vi "DEMO_04_WAVE_PRO.vi"() -> ()   [LabVIEW 2014]
uses:
  <vilib>/Instr/_visa.llb/VISA Configure Serial Port (Instr).vi
panel:
  in  "开始":bool
  in  "发送数据 3":bool
  in  "发送数据 2":bool
  in  "相位角 3":dbl
  in  "幅值 3":dbl
  in  "偏移 3":dbl
  in  "相位角 2":dbl
  in  "幅值 2":dbl
  in  "偏移 2":dbl
  in  "相位角":dbl
  in  "打开串口":bool
  in  "上位机控制":bool
  in  "停止传送":bool
  in  "开闭环":u16(ring) items=["  开环", "  闭环"]
  in  "幅值":dbl
  in  "频率":dbl
  in  "偏移":dbl
  in  "波形选择":u16(ring) items=["正弦波", "矩形波", "三角波", "锯齿波"]
  in  "发送数据":bool
  in  "波特率":u32(ring)=9600 items=["75"=75, "110"=110, "134"=134, "150"=150, "300"=300, "600"=600, "1200"=1200, "1800"=1800, "2400"=2400, "4800"=4800, "7200"=7200, "9600"=9600, "14400"=14400, "19200"=19200, "28800"=28800, "38400"=38400, "56000"=56000, "57600"=57600, "115200"=115200, "128000"=128000, "230400"=230400]
  in  "奇偶":enum16{"None", "Odd", "Even", "Mark", "Space"}(ring) caption="校验"
  in  "VISA资源名称":refnum<visa-resource-name>="COM1"
  # "发送相位角波形"
  # "下位机开闭环需要统一"
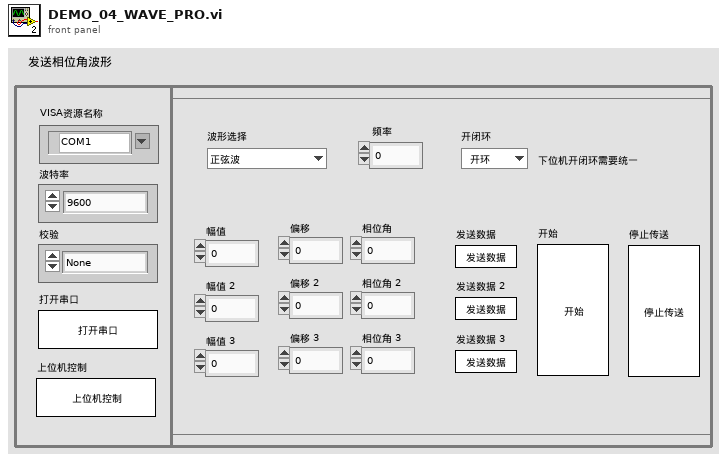
[diagram p1: front panel]
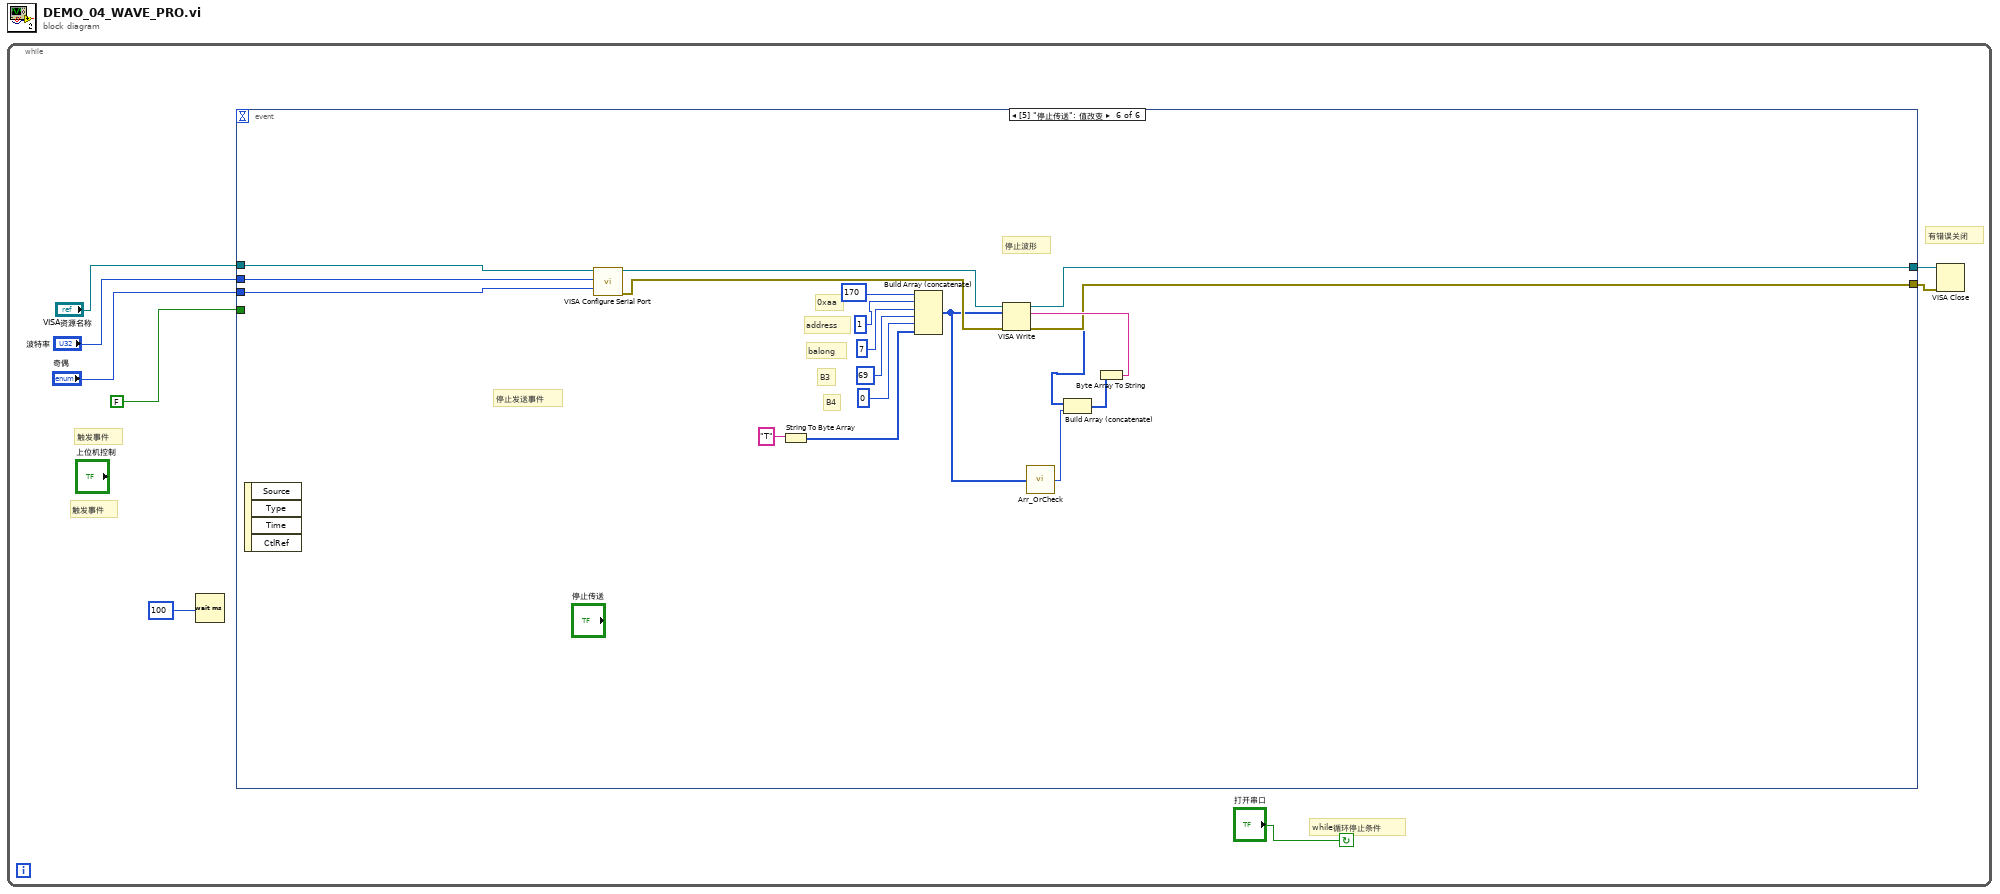
[diagram p0: block diagram]
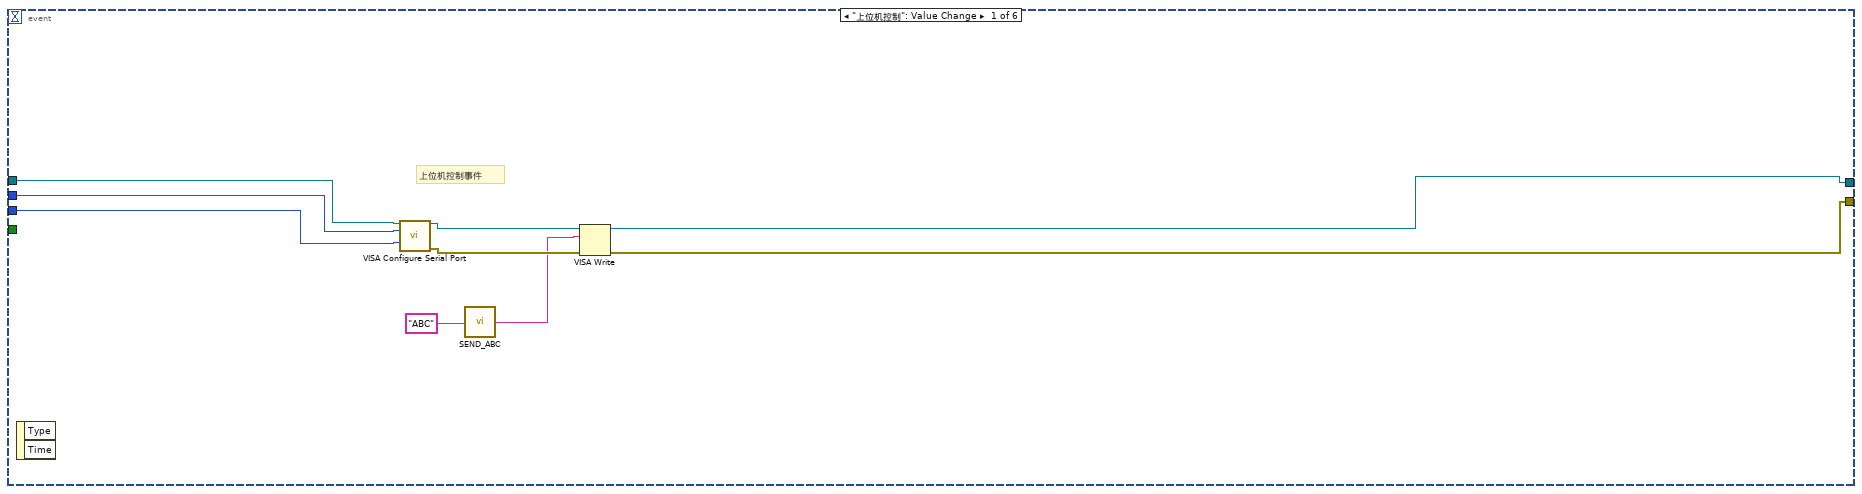
[diagram p2: hidden frame]
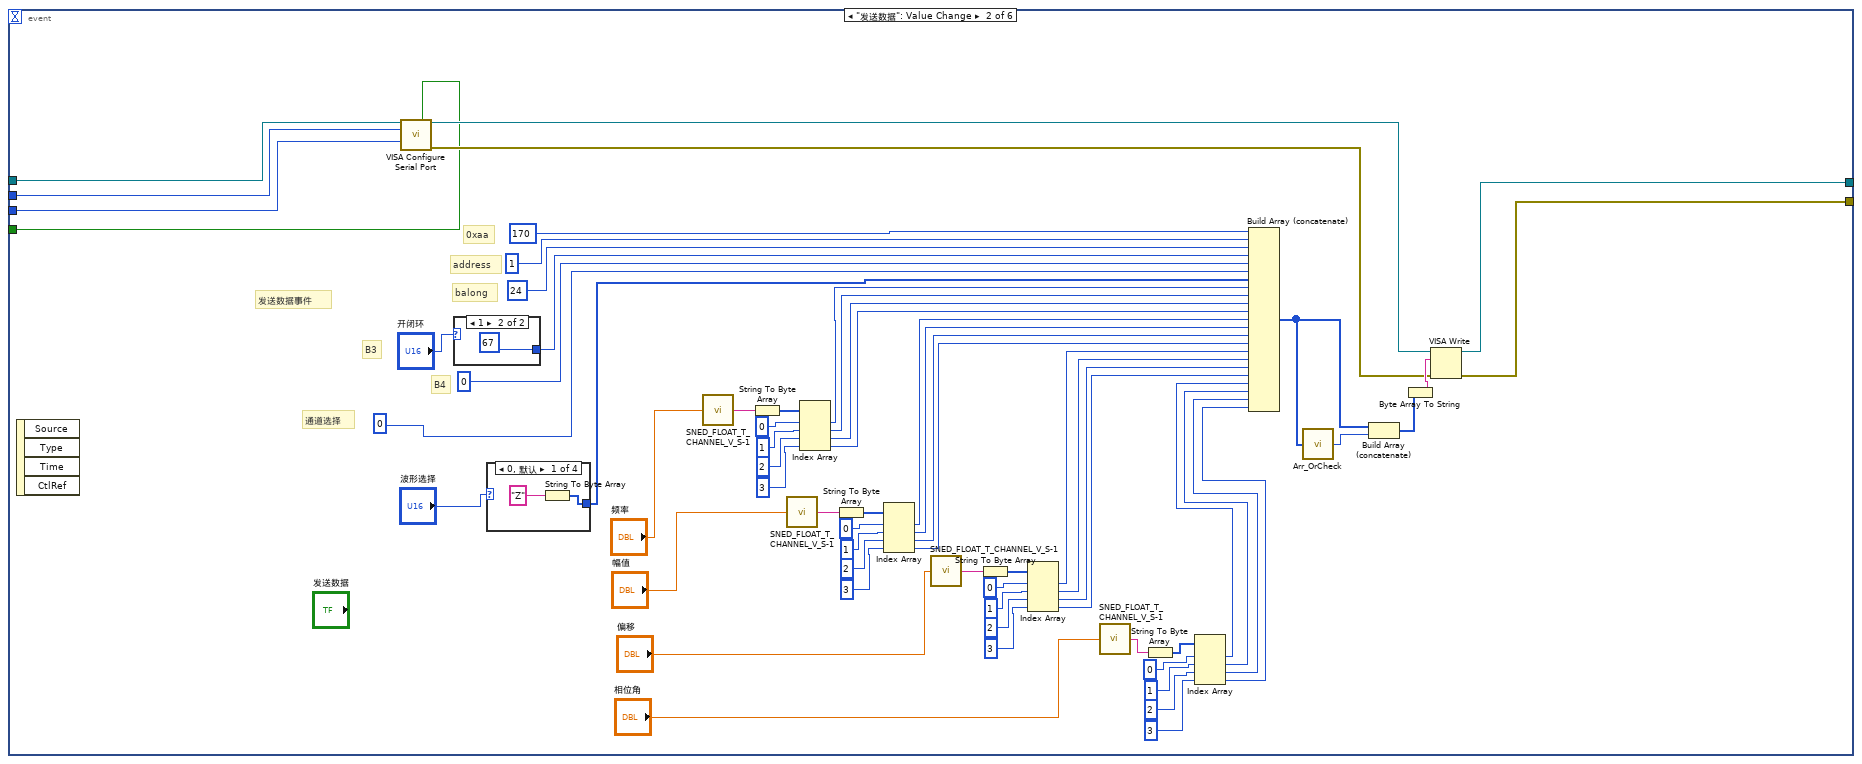
[diagram p3: hidden frame]
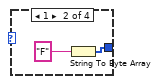
[diagram p4: hidden frame]
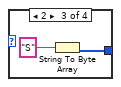
[diagram p5: hidden frame]
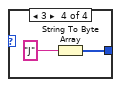
[diagram p6: hidden frame]
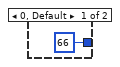
[diagram p7: hidden frame]
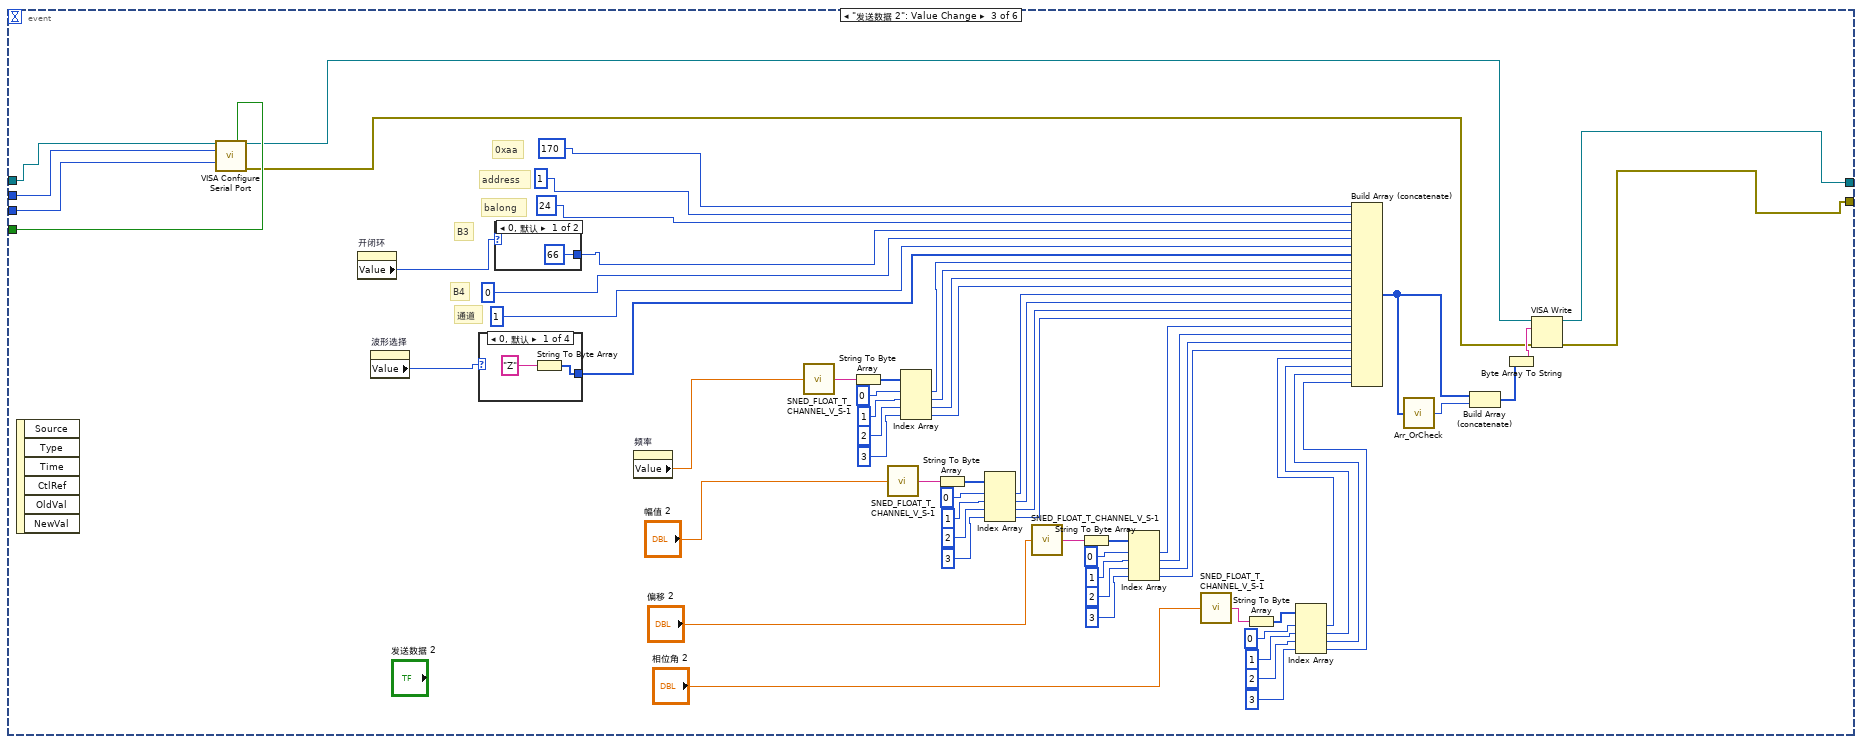
[diagram p8: hidden frame]
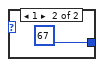
[diagram p9: hidden frame]
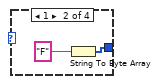
[diagram p10: hidden frame]
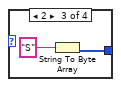
[diagram p11: hidden frame]
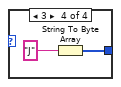
[diagram p12: hidden frame]
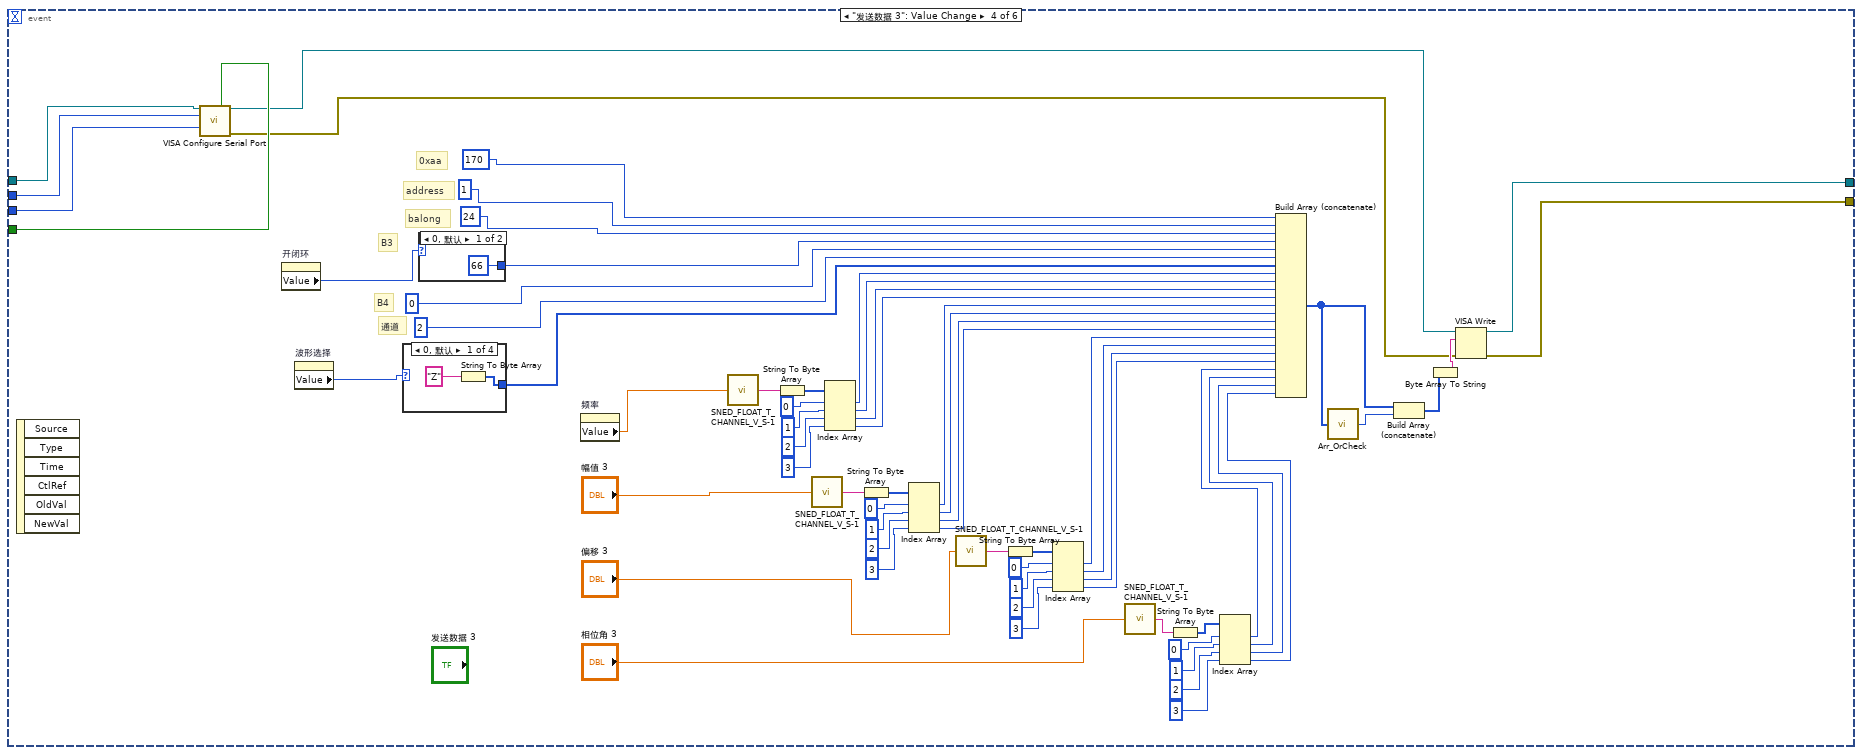
[diagram p13: hidden frame]
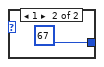
[diagram p14: hidden frame]
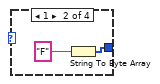
[diagram p15: hidden frame]
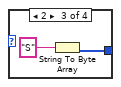
[diagram p16: hidden frame]
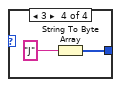
[diagram p17: hidden frame]
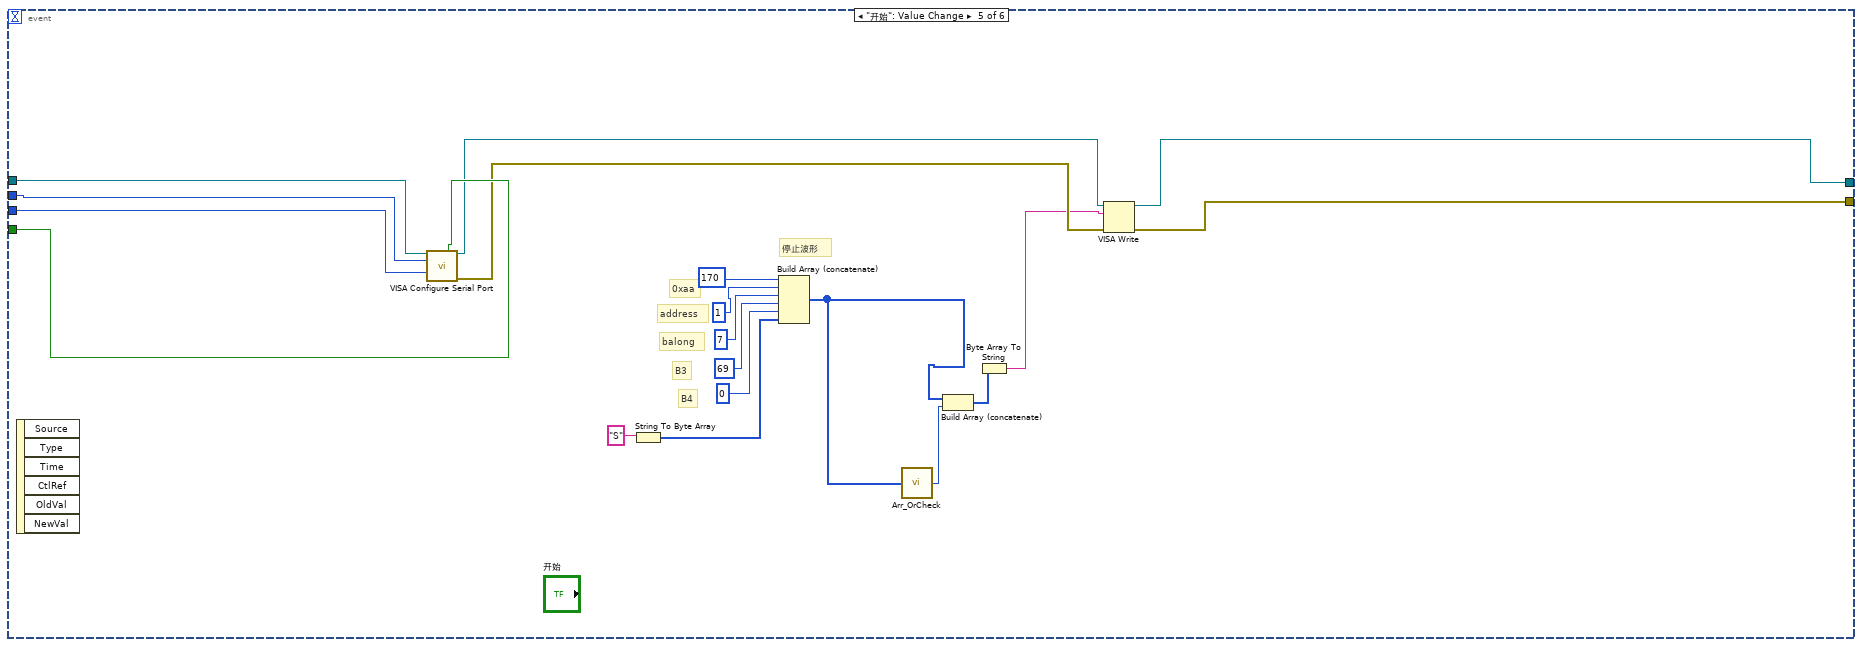
[diagram p18: hidden frame]
diagram:
  n1 = while {
    stop <- "打开串口" continue-if-true
    # "有错误关闭"
    # "while循环停止条件"
    # "触发事件"
    # "触发事件"
    n2 = Wait (ms)(milliseconds to wait=100) -> ()  [unwired: 1 out]
    n3 = event shown="[5] \"停止传送\": 值改变" {
      selector: _ -> [_ _ _ _ _ _]
      dyn-events: _ -> [_ _ _ _ _ _]
      timeout: _ -> [_ _ _ _ _ _]
      tunnel: "VISA资源名称" -> [w17 w35 w101 w177 w252 w279]
      tunnel: "波特率" -> [w16 w34 w100 w176 w251 w278]
      tunnel: "奇偶" -> [w15 w33 w99 w175 w250 w277]
      tunnel: [w10 w21 w94 w170 w245 w266] -> w3
      tunnel: [w9 w20 w95 w171 w244 w265] -> w2
      tunnel: FALSE -> [_ w19 w98 w174 w249 _]
      event "上位机控制": Value Change {
        # "上位机控制事件"
        n4 = event-data() -> ()  [unwired: 1 in, 2 out]
        n5 = call-poly "VISA Configure Serial Port"("VISA resource name"=w17, "baud rate (9600)"=w16, "parity (0:none)"=w15) -> ("VISA resource name out"=w14:refnum<visa-resource-name>, "error out"=w13:errorcluster)  [unwired: 11 in]
        n6 = call "SEND_ABC.vi"("SEND_ARR"="ABC") -> ("SEND_CHR"=w11:string)
        n7 = VISA Write(VISA resource name=w14, write buffer=w11, error in (no error)=w13) -> (VISA resource name out=w10:refnum<visa-resource-name>, error out=w9:errorcluster)  [unwired: 1 out]
      }
      event "发送数据": Value Change {
        # "通道选择"
        # "B4"
        # "B3"
        # "balong"
        # "address"
        # "0xaa"
        # "发送数据事件"
        n8 = event-data() -> ()  [unwired: 1 in, 4 out]
        n9 = call-poly "VISA Configure Serial Port"("VISA resource name"=w35, "Enable Termination\nChar (T)"=w19, "baud rate (9600)"=w34, "parity (0:none)"=w33) -> ("VISA resource name out"=w37:refnum<visa-resource-name>, "error out"=w36:errorcluster)  [unwired: 10 in]
        n10 = case shown="1" "开闭环" {
          tunnel: [66 67] -> w60
          frame 0, Default {
          }
          frame 1 {
          }
        }
        n11 = case shown="0, 默认" "波形选择" {
          tunnel: [w83 w85 w87 w89] -> w58
          frame 0, Default {
            n12 = String To Byte Array(string="Z") -> (unsigned byte array=w83:u8[])
          }
          frame 1 {
            n13 = String To Byte Array(string="F") -> (unsigned byte array=w85:u8[])
          }
          frame 2 {
            n14 = String To Byte Array(string="S") -> (unsigned byte array=w87:u8[])
          }
          frame 3 {
            n15 = String To Byte Array(string="J") -> (unsigned byte array=w89:u8[])
          }
        }
        n16 = call "SNED_FLOAT_T_CHANNEL_V_S-1.vi"("数据"="频率") -> ("字符串"=w81:string)
        n17 = String To Byte Array(string=w81) -> (unsigned byte array=w80:u8[])
        n18 = call "SNED_FLOAT_T_CHANNEL_V_S-1.vi"("数据"="幅值") -> ("字符串"=w75:string)
        n19 = Index Array(array=w80, index #1=0, index #2=1, index #3=2, index #4=3) -> (element #1=w54:u8, element #2=w53:u8, element #3=w52:u8, element #4=w51:u8)
        n20 = String To Byte Array(string=w75) -> (unsigned byte array=w74:u8[])
        n21 = Index Array(array=w74, index #1=0, index #2=1, index #3=2, index #4=3) -> (element #1=w50:u8, element #2=w49:u8, element #3=w48:u8, element #4=w47:u8)
        n22 = call "SNED_FLOAT_T_CHANNEL_V_S-1.vi"("数据"="偏移") -> ("字符串"=w69:string)
        n23 = String To Byte Array(string=w69) -> (unsigned byte array=w68:u8[])
        n24 = Index Array(array=w68, index #1=0, index #2=1, index #3=2, index #4=3) -> (element #1=w46:u8, element #2=w45:u8, element #3=w44:u8, element #4=w43:u8)
        n25 = call "SNED_FLOAT_T_CHANNEL_V_S-1.vi"("数据"="相位角") -> ("字符串"=w31:string)
        n26 = String To Byte Array(string=w31) -> (unsigned byte array=w30:u8[])
        n27 = Index Array(array=w30, index #1=0, index #2=1, index #3=2, index #4=3) -> (element #1=w25:u8, element #2=w24:u8, element #3=w23:u8, element #4=w22:u8)
        n28 = Build Array (concatenate)(170, 1, 24, w60, 0, 0, w58, w54, w53, w52, w51, w50, w49, w48, w47, w46, w45, w44, w43, w25, w24, w23, w22) -> (w42:i32[])
        n29 = call "Arr_OrCheck.vi"("数组"=w42) -> ("抑或的数据值"=w41:u8)
        n30 = Build Array (concatenate)(w42, w41) -> (w40:i32[])
        n31 = Byte Array To String(unsigned byte array=w40) -> (string=w39:string)
        n32 = VISA Write(VISA resource name=w37, write buffer=w39, error in (no error)=w36) -> (VISA resource name out=w21:refnum<visa-resource-name>, error out=w20:errorcluster)  [unwired: 1 out]
      }
      event "发送数据 2": Value Change {
        # "通道"
        # "B4"
        # "B3"
        # "balong"
        # "address"
        # "0xaa"
        n33 = event-data() -> ()  [unwired: 1 in, 6 out]
        n34 = call-poly "VISA Configure Serial Port"("VISA resource name"=w101, "Enable Termination\nChar (T)"=w98, "baud rate (9600)"=w100, "parity (0:none)"=w99) -> ("VISA resource name out"=w97:refnum<visa-resource-name>, "error out"=w96:errorcluster)  [unwired: 10 in]
        n35 = property on="开闭环" class="Ring (严格)"() -> ("Value"=w113:u16)  [unwired: 2 in, 2 out]
        n36 = property on="波形选择" class="Ring (严格)"() -> ("Value"=w112:u16)  [unwired: 2 in, 2 out]
        n37 = case shown="0, 默认" w112 {
          tunnel: [w160 w162 w164 w166] -> w111
          frame 0, Default {
            n38 = String To Byte Array(string="Z") -> (unsigned byte array=w160:u8[])
          }
          frame 1 {
            n39 = String To Byte Array(string="F") -> (unsigned byte array=w162:u8[])
          }
          frame 2 {
            n40 = String To Byte Array(string="S") -> (unsigned byte array=w164:u8[])
          }
          frame 3 {
            n41 = String To Byte Array(string="J") -> (unsigned byte array=w166:u8[])
          }
        }
        n42 = case shown="0, 默认" w113 {
          tunnel: [66 67] -> w108
          frame 0, Default {
          }
          frame 1 {
          }
        }
        n43 = property on="频率" class="DigNum (严格)"() -> ("Value"=w93:dbl)  [unwired: 2 in, 2 out]
        n44 = call "SNED_FLOAT_T_CHANNEL_V_S-1.vi"("数据"=w93) -> ("字符串"=w157:string)
        n45 = String To Byte Array(string=w157) -> (unsigned byte array=w156:u8[])
        n46 = call "SNED_FLOAT_T_CHANNEL_V_S-1.vi"("数据"="幅值 2") -> ("字符串"=w151:string)
        n47 = Index Array(array=w156, index #1=0, index #2=1, index #3=2, index #4=3) -> (element #1=w139:u8, element #2=w138:u8, element #3=w137:u8, element #4=w136:u8)
        n48 = String To Byte Array(string=w151) -> (unsigned byte array=w150:u8[])
        n49 = Index Array(array=w150, index #1=0, index #2=1, index #3=2, index #4=3) -> (element #1=w135:u8, element #2=w134:u8, element #3=w133:u8, element #4=w132:u8)
        n50 = call "SNED_FLOAT_T_CHANNEL_V_S-1.vi"("数据"="偏移 2") -> ("字符串"=w145:string)
        n51 = String To Byte Array(string=w145) -> (unsigned byte array=w144:u8[])
        n52 = Index Array(array=w144, index #1=0, index #2=1, index #3=2, index #4=3) -> (element #1=w131:u8, element #2=w130:u8, element #3=w129:u8, element #4=w128:u8)
        n53 = call "SNED_FLOAT_T_CHANNEL_V_S-1.vi"("数据"="相位角 2") -> ("字符串"=w123:string)
        n54 = String To Byte Array(string=w123) -> (unsigned byte array=w122:u8[])
        n55 = Index Array(array=w122, index #1=0, index #2=1, index #3=2, index #4=3) -> (element #1=w117:u8, element #2=w116:u8, element #3=w115:u8, element #4=w114:u8)
        n56 = Build Array (concatenate)(170, 1, 24, w108, 0, 1, w111, w139, w138, w137, w136, w135, w134, w133, w132, w131, w130, w129, w128, w117, w116, w115, w114) -> (w127:i32[])
        n57 = call "Arr_OrCheck.vi"("数组"=w127) -> ("抑或的数据值"=w126:u8)
        n58 = Build Array (concatenate)(w127, w126) -> (w125:i32[])
        n59 = Byte Array To String(unsigned byte array=w125) -> (string=w124:string)
        n60 = VISA Write(VISA resource name=w97, write buffer=w124, error in (no error)=w96) -> (VISA resource name out=w94:refnum<visa-resource-name>, error out=w95:errorcluster)  [unwired: 1 out]
      }
      event "发送数据 3": Value Change {
        # "通道"
        # "B4"
        # "B3"
        # "balong"
        # "address"
        # "0xaa"
        n61 = event-data() -> ()  [unwired: 1 in, 6 out]
        n62 = call-poly "VISA Configure Serial Port"("VISA resource name"=w177, "Enable Termination\nChar (T)"=w174, "baud rate (9600)"=w176, "parity (0:none)"=w175) -> ("VISA resource name out"=w173:refnum<visa-resource-name>, "error out"=w172:errorcluster)  [unwired: 10 in]
        n63 = property on="开闭环" class="Ring (严格)"() -> ("Value"=w189:u16)  [unwired: 2 in, 2 out]
        n64 = property on="波形选择" class="Ring (严格)"() -> ("Value"=w188:u16)  [unwired: 2 in, 2 out]
        n65 = case shown="0, 默认" w188 {
          tunnel: [w235 w237 w239 w241] -> w187
          frame 0, Default {
            n66 = String To Byte Array(string="Z") -> (unsigned byte array=w235:u8[])
          }
          frame 1 {
            n67 = String To Byte Array(string="F") -> (unsigned byte array=w237:u8[])
          }
          frame 2 {
            n68 = String To Byte Array(string="S") -> (unsigned byte array=w239:u8[])
          }
          frame 3 {
            n69 = String To Byte Array(string="J") -> (unsigned byte array=w241:u8[])
          }
        }
        n70 = case shown="0, 默认" w189 {
          tunnel: [66 67] -> w169
          frame 0, Default {
          }
          frame 1 {
          }
        }
        n71 = property on="频率" class="DigNum (严格)"() -> ("Value"=w181:dbl)  [unwired: 2 in, 2 out]
        n72 = call "SNED_FLOAT_T_CHANNEL_V_S-1.vi"("数据"=w181) -> ("字符串"=w232:string)
        n73 = String To Byte Array(string=w232) -> (unsigned byte array=w231:u8[])
        n74 = call "SNED_FLOAT_T_CHANNEL_V_S-1.vi"("数据"="幅值 3") -> ("字符串"=w226:string)
        n75 = Index Array(array=w231, index #1=0, index #2=1, index #3=2, index #4=3) -> (element #1=w168:u8, element #2=w214:u8, element #3=w213:u8, element #4=w212:u8)
        n76 = String To Byte Array(string=w226) -> (unsigned byte array=w225:u8[])
        n77 = Index Array(array=w225, index #1=0, index #2=1, index #3=2, index #4=3) -> (element #1=w211:u8, element #2=w210:u8, element #3=w209:u8, element #4=w208:u8)
        n78 = call "SNED_FLOAT_T_CHANNEL_V_S-1.vi"("数据"="偏移 3") -> ("字符串"=w220:string)
        n79 = String To Byte Array(string=w220) -> (unsigned byte array=w219:u8[])
        n80 = Index Array(array=w219, index #1=0, index #2=1, index #3=2, index #4=3) -> (element #1=w207:u8, element #2=w206:u8, element #3=w205:u8, element #4=w204:u8)
        n81 = call "SNED_FLOAT_T_CHANNEL_V_S-1.vi"("数据"="相位角 3") -> ("字符串"=w199:string)
        n82 = String To Byte Array(string=w199) -> (unsigned byte array=w198:u8[])
        n83 = Index Array(array=w198, index #1=0, index #2=1, index #3=2, index #4=3) -> (element #1=w193:u8, element #2=w192:u8, element #3=w191:u8, element #4=w190:u8)
        n84 = Build Array (concatenate)(170, 1, 24, w169, 0, 2, w187, w168, w214, w213, w212, w211, w210, w209, w208, w207, w206, w205, w204, w193, w192, w191, w190) -> (w203:i32[])
        n85 = call "Arr_OrCheck.vi"("数组"=w203) -> ("抑或的数据值"=w202:u8)
        n86 = Build Array (concatenate)(w203, w202) -> (w201:i32[])
        n87 = Byte Array To String(unsigned byte array=w201) -> (string=w200:string)
        n88 = VISA Write(VISA resource name=w173, write buffer=w200, error in (no error)=w172) -> (VISA resource name out=w170:refnum<visa-resource-name>, error out=w171:errorcluster)  [unwired: 1 out]
      }
      event "开始": Value Change {
        # "停止波形"
        # "B4"
        # "B3"
        # "balong"
        # "address"
        # "0xaa"
        n89 = event-data() -> ()  [unwired: 1 in, 6 out]
        n90 = call-poly "VISA Configure Serial Port"("VISA resource name"=w252, "Enable Termination\nChar (T)"=w249, "baud rate (9600)"=w251, "parity (0:none)"=w250) -> ("VISA resource name out"=w248:refnum<visa-resource-name>, "error out"=w247:errorcluster)  [unwired: 10 in]
        n91 = String To Byte Array(string="S") -> (unsigned byte array=w253:u8[])
        n92 = Build Array (concatenate)(170, 1, 7, 69, 0, w253) -> (w243:i32[])
        n93 = call "Arr_OrCheck.vi"("数组"=w243) -> ("抑或的数据值"=w260:u8)
        n94 = Build Array (concatenate)(w243, w260) -> (w261:i32[])
        n95 = Byte Array To String(unsigned byte array=w261) -> (string=w246:string)
        n96 = VISA Write(VISA resource name=w248, write buffer=w246, error in (no error)=w247) -> (VISA resource name out=w245:refnum<visa-resource-name>, error out=w244:errorcluster)  [unwired: 1 out]
      }
      event "停止传送": Value Change {
        # "停止波形"
        # "B4"
        # "B3"
        # "balong"
        # "address"
        # "0xaa"
        # "停止发送事件"
        n97 = event-data() -> ()  [unwired: 1 in, 4 out]
        n98 = call-poly "VISA Configure Serial Port"("VISA resource name"=w279, "baud rate (9600)"=w278, "parity (0:none)"=w277) -> ("VISA resource name out"=w268:refnum<visa-resource-name>, "error out"=w267:errorcluster)  [unwired: 11 in]
        n99 = String To Byte Array(string="T") -> (unsigned byte array=w263:u8[])
        n100 = Build Array (concatenate)(170, 1, 7, 69, 0, w263) -> (w262:i32[])
        n101 = call "Arr_OrCheck.vi"("数组"=w262) -> ("抑或的数据值"=w274:u8)
        n102 = Build Array (concatenate)(w262, w274) -> (w275:i32[])
        n103 = Byte Array To String(unsigned byte array=w275) -> (string=w276:string)
        n104 = VISA Write(VISA resource name=w268, write buffer=w276, error in (no error)=w267) -> (VISA resource name out=w266:refnum<visa-resource-name>, error out=w265:errorcluster)  [unwired: 1 out]
      }
    }
    n105 = VISA Close(VISA resource name=w3, error in (no error)=w2) -> ()  [unwired: 1 out]
  }
